vi "StandardizeComicTitle.vi"(5 "make sortable (F)":bool, 7 "extention (\"\"=none)":string=".cbz", 11 "title in":string) -> (3 "title out":string)   [LabVIEW 2024]
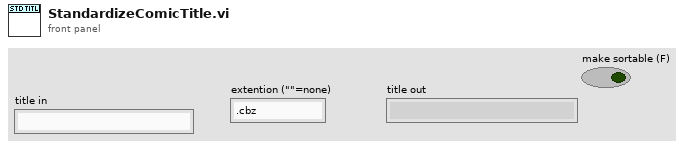
[diagram p1: front panel]
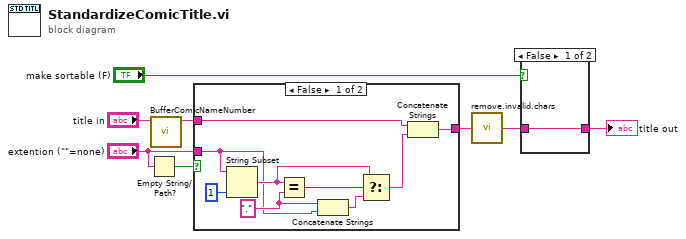
[diagram p0: block diagram]
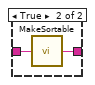
[diagram p3: hidden frame]
diagram:
  n1 = Empty String/Path?(string/path="extention (\"\"=none)") -> (empty?=w7:bool)
  n2 = call "BufferComicNameNumber.vi"("string in"="title in") -> ("buffered number string"=w6:string)  [unwired: 10 in]
  n3 = case shown="False" w7 {
    tunnel: w6 -> [w16 w18]
    tunnel: [w17 w18] -> w5
    tunnel: "extention (\"\"=none)" -> [w9 _]
    frame False {
      w12 = "." ("y")
      n4 = String Subset(string=w9, length (rest)=1 ("length (rest)")) -> (substring=w11:string)  [unwired: 1 in]
      n5 = Equal?(x=w11, y=w12) -> (x = y?=w14:bool)
      n6 = Concatenate Strings(w12, w9) -> (w13:string)
      n7 = Select(t=w11, s=w14, f=w13) -> (s? t:f=w10:string)
      n8 = Concatenate Strings(w16, w10) -> (w17:string)
    }
    frame True {
    }
  }
  n9 = call "remove.invalid.chars.vi"("string in"=w5) -> ("string out"=w2:string)
  n10 = case shown="False" "make sortable (F)" {
    tunnel: w2 -> [w19 w21]
    tunnel: [w19 w20] -> w1
    frame False {
    }
    frame True {
      n11 = call "MakeSortable.vi"("string in"=w21) -> ("string out"=w20:string)
    }
  }
  "title out" <- w1
